vi "Write model.vi"(10 "Model.lvlib:Model.lvclass":refnum<class "IModel.lvclass">, 11 "ConcreteContext1 in":refnum<class "ContextThisComponent.lvclass">) -> (3 "ConcreteContext1 out":refnum<class "ContextThisComponent.lvclass">)   [LabVIEW 2012, in "ContextThisComponent.lvclass"]
uses:
  ContextThisComponent.lvclass
  IModel/IModel.lvclass
  ContextThisComponent.lvclass/ContextThisComponent.ctl
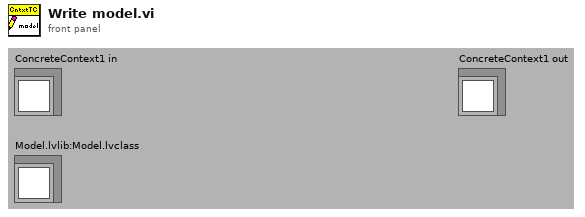
[diagram p1: front panel]
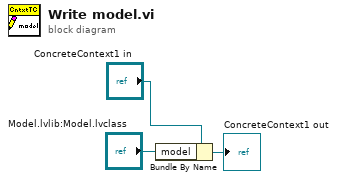
[diagram p0: block diagram]
diagram:
  n1 = Bundle By Name(cluster="ConcreteContext1 in", "model"="Model.lvlib:Model.lvclass") -> (→"ConcreteContext1 out":refnum<class "ContextThisComponent.lvclass">)
